vi "ReleaseQueues.vi"(8 "error in (no error)":errorcluster, 11 "DAQmx":refnum<class "DAQmx.lvclass">) -> (0 "error out":errorcluster, 3 "DAQmx out":refnum<class "DAQmx.lvclass">)   [LabVIEW 2019, in "DAQmx.lvclass"]
uses:
  DAQmx.lvclass
  DAQmx.lvclass/DAQmx.ctl
panel:
  # "For instructions on how to use the JKI State Machine Objects, examples and video tutorials, visit:\nhttp://jki.net/state-machine-objects/\n\nJKI State Machine Objects™\nhttp://jki.net/state-machine-objects/\nCopyright (C) 2005-2015, JKI <info@jki.net>\nALL RIGHTS RESERVED"
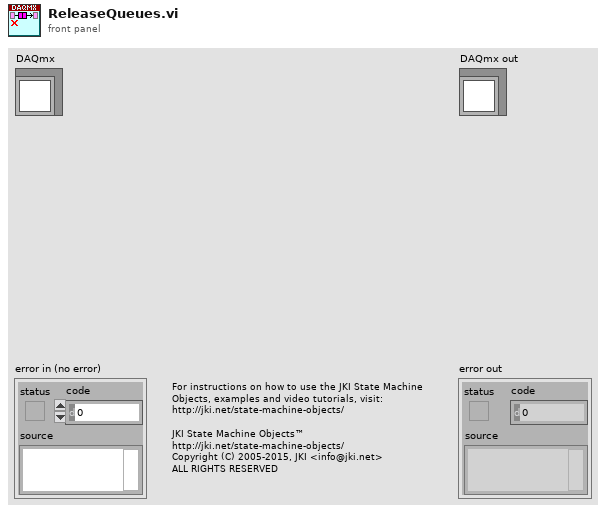
[diagram p1: front panel]
types:
  T1 = typedef "DAQmx.lvclass/PrivateQueues--Cluster.ctl" = cluster{"Action":refnum<queue>, "Timing":refnum<queue>, "AOconfig":refnum<queue>, "AIconfig":refnum<queue>}
  T2 = typedef "DAQmx.lvclass/PublicQueues--Cluster.ctl" = cluster{"AOwfm":refnum<queue>}
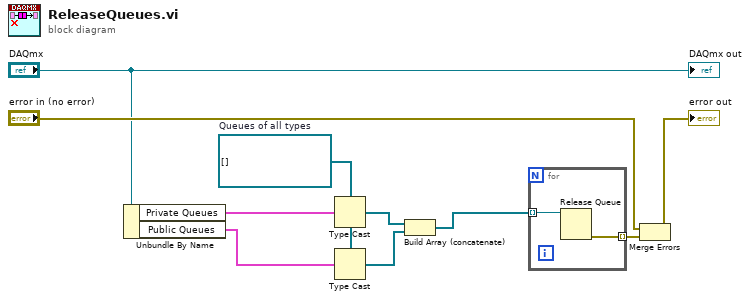
[diagram p0: block diagram]
diagram:
  w1 = refnum<queue>[] []  # Queues of all types
  n1 = Unbundle By Name("DAQmx") -> ("Private Queues"=w8:T1, "Public Queues"=w5:T2)
  n2 = Type Cast(type=w1, x=w8) -> (*(type *) &x=w3:refnum<queue>[])
  n3 = Type Cast(type=w1, x=w5) -> (*(type *) &x=w4:refnum<queue>[])
  n4 = Build Array (concatenate)(w3, w4) -> (w2:refnum<queue>[])
  n5 = for {
    tunnel: w2 -> [w11] mode=indexing
    tunnel: [w12] -> w10 mode=indexing
    n6 = Release Queue(queue=w11) -> (error out=w12:errorcluster)  [unwired: 2 in, 2 out]
  }
  n7 = Merge Errors("error in (no error)", w10) -> (→"error out":errorcluster)
  "DAQmx out" <- "DAQmx"
